vi "Read Scale.vi"(8 "error in (no error)":errorcluster, 11 "MFC in":refnum<class "Scale.lvclass">) -> (0 "error out":errorcluster, 3 "MFC out":refnum<class "Scale.lvclass">)   [LabVIEW 2013, in "Scale.lvlib" / "Scale.lvclass"]
uses:
  Scale.lvclass
  Scale.lvclass/Scale.ctl
  Read VISA.vi
  Read Value.vi
  PluginInterface/PluginInterface.lvlibp/PluginInterfaceClass/Read DVR.vi
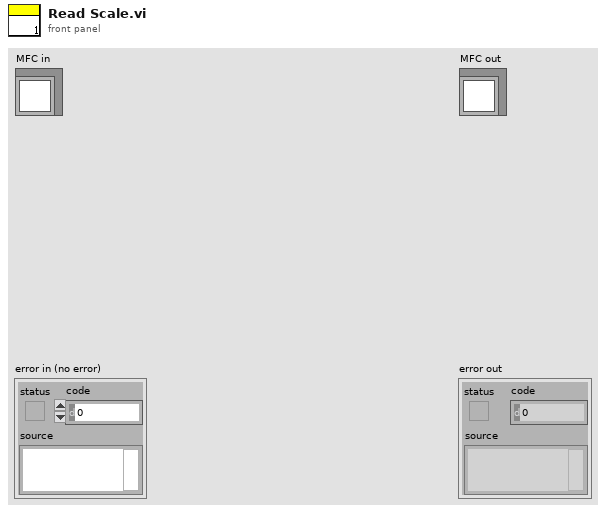
[diagram p1: front panel]
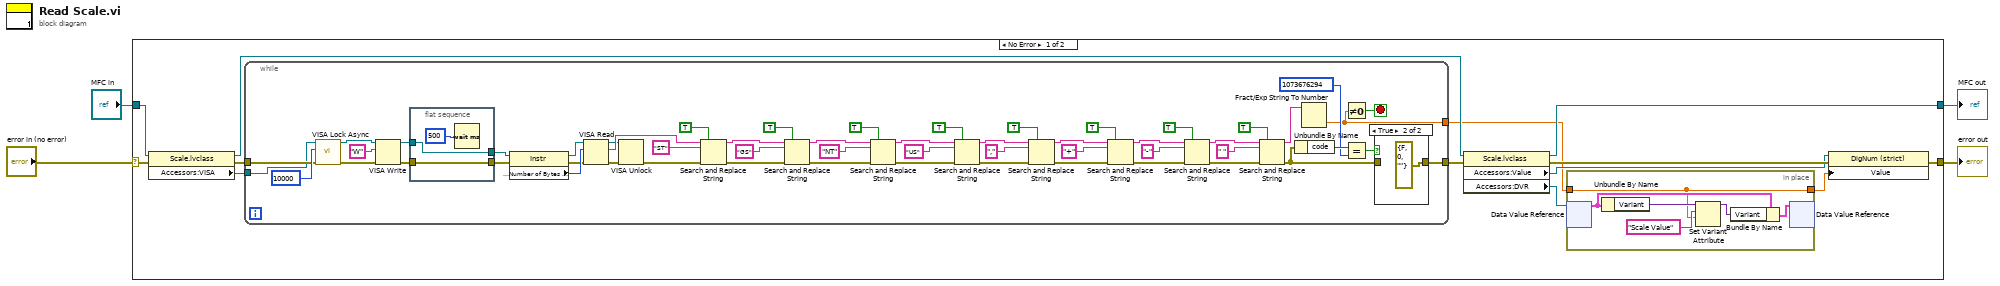
[diagram p0: block diagram]
diagram:
  n1 = case shown="No Error" "error in (no error)" {
    selector: "error in (no error)" -> [w16 w85]
    tunnel: [w5 w85] -> w3
    tunnel: [w14 w84] -> w1
    tunnel: "MFC in" -> [w17 w84]
    frame No Error {
      n2 = property class="Scale.lvclass"(reference=w17, error in=w16) -> (reference out=w7:refnum<class "Scale.lvclass">, error out=w10:errorcluster, "Accessors:VISA"=w9:refnum<visa-resource-name>)
      n3 = while {
        tunnel: [w19] -> w8
        tunnel: w10 -> [w21]
        tunnel: w9 -> [w20]
        tunnel: [w18] -> w6
        stop <- w22 stop-if-true
        n4 = call <vilib>:"VISA Lock Async.vi"("error in (no error)"=w21, "timeout (0)"=u32 10000, "VISA resource name"=w20) -> ("error out"=w26:errorcluster, "VISA resource name out"=w27:refnum<visa-resource-name>)  [unwired: 6 in, 1 out]
        n5 = VISA Write(VISA resource name=w27, write buffer="W", error in (no error)=w26) -> (VISA resource name out=w68:refnum<visa-resource-name>, error out=w67:errorcluster)  [unwired: 1 out]
        n6 = flat-sequence {
          tunnel: w68 -> [w75]
          tunnel: [w75] -> w62
          tunnel: [w74] -> w66
          tunnel: w67 -> [w74]
          frame #0 {
            n7 = Wait (ms)(milliseconds to wait=u32 500 ("ms before read")) -> ()  [unwired: 1 out]
          }
        }
        n8 = property class="Instr"(reference=w62, error in=w66) -> (reference out=w65:refnum<visa-resource-name>, error out=w63:errorcluster, "Serial Settings:Number of Bytes at Serial Port"=w64:u32)
        n9 = VISA Read(VISA resource name=w65, byte count=w64, error in (no error)=w63) -> (VISA resource name out=w25:refnum<visa-resource-name>, read buffer=w30:string, error out=w24:errorcluster)  [unwired: 1 out]
        n10 = VISA Unlock(8:w24, 11:w25) -> (0:w23:errorcluster)  [unwired: 1 out]
        n11 = Search and Replace String(replace all?=TRUE ("replace all? (F)"), input string=w30, search string="ST" ("input string"), error in=w23) -> (result string=w56:string, error out=w51:errorcluster)  [unwired: 4 in, 2 out]
        n12 = Search and Replace String(replace all?=TRUE ("replace all? (F)"), input string=w56, search string="GS" ("input string"), error in=w51) -> (result string=w55:string, error out=w52:errorcluster)  [unwired: 4 in, 2 out]
        n13 = Search and Replace String(replace all?=TRUE ("replace all? (F)"), input string=w55, search string="NT" ("input string"), error in=w52) -> (result string=w54:string, error out=w53:errorcluster)  [unwired: 4 in, 2 out]
        n14 = Search and Replace String(replace all?=TRUE ("replace all? (F)"), input string=w54, search string="US" ("input string"), error in=w53) -> (result string=w38:string, error out=w41:errorcluster)  [unwired: 4 in, 2 out]
        n15 = Search and Replace String(replace all?=TRUE ("replace all? (F)"), input string=w38, search string="," ("input string"), error in=w41) -> (result string=w37:string, error out=w40:errorcluster)  [unwired: 4 in, 2 out]
        n16 = Search and Replace String(replace all?=TRUE ("replace all? (F)"), input string=w37, search string="+" ("input string"), error in=w40) -> (result string=w36:string, error out=w39:errorcluster)  [unwired: 4 in, 2 out]
        n17 = Search and Replace String(replace all?=TRUE ("replace all? (F)"), input string=w36, search string="-" ("input string"), error in=w39) -> (result string=w33:string, error out=w32:errorcluster)  [unwired: 4 in, 2 out]
        n18 = Search and Replace String(replace all?=TRUE ("replace all? (F)"), input string=w33, search string=" " ("input string"), error in=w32) -> (result string=w31:string, error out=w29:errorcluster)  [unwired: 4 in, 2 out]
        n19 = Unbundle By Name(w29) -> ("code"=w72:i32)
        n20 = Fract/Exp String To Number(string=w31) -> (number=w18:dbl)  [unwired: 3 in, 1 out]
        n21 = Not Equal To 0?(x=w18) -> (x != 0?=w22:bool)
        n22 = Equal?(x=w72, y=1073676294) -> (x = y?=w70:bool)
        n23 = case shown="True" w70 {
          tunnel: w29 -> [w76 _]
          tunnel: [w76 errorcluster {"status"=FALSE, "code"=0, "source"=""} ("error constant")] -> w19
          frame False {
          }
          frame True {
          }
        }
      }
      n24 = property class="Scale.lvclass"(reference=w7, error in=w8) -> (reference out=w14:refnum<class "Scale.lvclass">, error out=w15:errorcluster, "Accessors:Value"=w12:refnum<vi>, "Accessors:DVR"=w13:refnum<data-value>)
      n25 = in-place {
        in-place-border: w6 -> [w78]
        in-place-border: [w78] -> w11
        n26 = in-place-dvr #1(w13) -> (w80:cluster{"Array":string[], "Variant":variant})  [unwired: 1 out]
        n27 = Unbundle By Name(w80) -> ("Variant"=w82:variant)
        n28 = Set Variant Attribute(Variant=w82, name="Scale Value", value=w78) -> (Variant out=w81:variant)  [unwired: 1 in, 2 out]
        n29 = Bundle By Name(cluster=w80, "Variant"=w81) -> (w83:cluster{"Array":string[], "Variant":variant})
        n30 = in-place-dvr #1(w83) -> ()  [unwired: 2 out]
      }
      n31 = property class="DigNum (strict)"(reference=w12, error in=w15, "Value"=w11) -> (error out=w5:errorcluster)  [unwired: 1 out]
    }
    frame Error {
    }
  }
  "error out" <- w3
  "MFC out" <- w1
